vi "MasterAcquisitionFile_IOS.vi"() -> ()   [LabVIEW 2020]
uses:
  <vilib>/vision/driver/IMAQdx.llb/IMAQdx Camera Control Mode.ctl
  <vilib>/vision/driver/IMAQdx.llb/IMAQdx Acquisition Mode.ctl
  <vilib>/userDefined/High Color/IMAQdx.ctl
  <vilib>/vision/driver/IMAQdx.llb/IMAQdx Buffer Number Mode.ctl
  <vilib>/DAQmx/write.llb/DAQmx Write (Digital 1D Wfm NChan NSamp).vi
  <vilib>/DAQmx/read.llb/DAQmx Read (Analog 1D Wfm NChan NSamp).vi
  <vilib>/Waveform/DWDTOps.llb/DWDT Digital to Boolean Array.vi
  <vilib>/DAQmx/create/channels.llb/DAQmx Create Channel (CO-Pulse Generation-Frequency).vi
  <vilib>/DAQmx/configure/timing.llb/DAQmx Timing (Implicit).vi
  <vilib>/DAQmx/create/channels.llb/DAQmx Create Channel (AI-Voltage-Basic).vi
  <vilib>/DAQmx/configure/timing.llb/DAQmx Timing (Sample Clock).vi
  <vilib>/DAQmx/configure/trigger.llb/DAQmx Start Trigger (Digital Edge).vi
  <vilib>/DAQmx/create/channels.llb/DAQmx Create Channel (DO-Digital Output).vi
  <vilib>/Waveform/DWDTOps.llb/DWDT Boolean Array to Digital.vi
  <vilib>/Waveform/DWDTOps.llb/DWDT Uncompress Digital.vi
  <vilib>/DAQmx/miscellaneous.llb/DAQmx Fill In Error Info.vi
  <vilib>/vision/driver/NI_Vision_Acquisition_Software.lvlib
  <resource>/objmgr/imaqdx.rc
  <resource>/objmgr/daqmx.rc
panel:
  out "LED":bool
  out "Auditory":bool
  out "RPad":bool
  out "LPad":bool
  out "Finished":bool
  in  "Generate Stimuli":bool=TRUE
  in  "Sol Stim Parameters":cluster{"Fs":dbl, "Samples":dbl}
  in  "LED Stim Parameters":cluster{"Fs":dbl, "Samples":dbl}
  in  "Sol Duty Cycle (%)":dbl=10.0
  in  "Sol Freq":dbl=1.0
  in  "Sol Dur (s)":dbl=1.0
  in  "LED Duty Cycle (%)":dbl=10.0
  in  "LED Freq":dbl=10.0
  in  "LED Dur (s)":dbl=2.0
  out "Stimulus Order":digitalwaveform[](graph)=[{"t0"=timestamp(0 s since 1904-01-01), "dt"=5e-05, "Y"={"transitions"=[], "data"=array18001000x1[18001000 elements]}}, {"t0"=timestamp(0 s since 1904-01-01), "dt"=5e-05, "Y"={"transitions"=[], "data"=array18001000x1[18001000 elements]}}, {"t0"=timestamp(0 s since 1904-01-01), "dt"=5e-05, "Y"={"transitions"=[], "data"=array18001000x1[18001000 elements]}}, {"t0"=timestamp(0 s since 1904-01-01), "dt"=5e-05, "Y"={"transitions"=[], "data"=array18001000x1[18001000 elements]}}]
  out "Solenoid Stim":digitalwaveform(graph)={"t0"=timestamp(0 s since 1904-01-01), "dt"=5e-05, "Y"={"transitions"=[], "data"=array100000x1[100000 elements]}}
  in  "Trial Offset (s)":dbl=15.0
  in  "Interstim (s)":dbl=30.0
  in  "Right Pad":dbl=1.0
  in  "Left Pad":dbl=1.0
  in  "Auditory":dbl=1.0
  in  "LED":dbl
  out "?":T1(plugin-control)
  out "?":T1(plugin-control)
  out "?":T1(plugin-control)
  out "?":T1(plugin-control)
  in  "stop":bool
  out "CBV Cam":bool=TRUE
  out "Pupil Cam":bool=TRUE
  out "Whisk Cam":bool=TRUE
  out "Web Cam":bool=TRUE
  out "Analog":bool=TRUE
  out "Web Cam Fs":dbl(knob)=29.946097025354362 scale=0.0..200.0
  out "CBV Cam Fs":dbl(knob)=30.0 scale=0.0..200.0
  out "Whisk Cam Fs":dbl(knob)=150.04985044865404 scale=0.0..200.0
  out "Last Whisk\nBuffer 2":u32=16153
  out "Pupil Cam Fs":dbl(knob)=30.00491883915396 scale=0.0..200.0
  out "Dropped 2":u32(slide) caption="Pupil Cam" scale=0.0..99.0
  in  "Exposure Time (microsec)":string="10000"
  out "Dev1 Samples":i32=10769152
  in  "Dev1 Analog Channels":string[](array[string])=["Cortical_LH", "Force_Sensor", "LPadSol", "RPadSol", "AudSol", "Hippocampus", "EMG", "Cortical_RH", "OptoLED"]
  in  "Analog Acquisition":cluster{"Analog Fs":u16}={"Analog Fs"=20000} {"Analog Fs" format="%0.0f"}
  in  "Sampling Rates":T2={"CBV Cam Fs"=30, "Whisk Cam Fs"=150, "Web Cam Fs"=15, "Pupil Cam Fs"=30}
  out "Notes Size":i32=8
  out "Notes Reversed":string[](array[string])=["Experimenter", "Animal ID", "Hemisphere", "Solenoid PSI", "Isoflurane time", "Session ID", "Amplifier Gain", "LED power (mW)"]
  out "Notes Array":string[](array[string])=["LED power (mW)", "Amplifier Gain", "Session ID", "Isoflurane time", "Solenoid PSI", "Hemisphere", "Animal ID", "Experimenter"]
  in  "Notes:":T3={"Experimenter"="Kevin", "Animal ID"="T220", "Hemisphere"="Both", "Solenoid PSI"="10", "Isoflurane time"="1000", "Session ID"="Imaging Session One", "Amplifier Gain"="10000", "LED power (mW)"="10"}
  in  "Target Path":path=path "D:/T220/Imaging Session One - 17 May 2021" caption="Final Save Location"
  out "Dropped":u32(slide) caption="Whisk Cam" scale=0.0..999.0
  out "Filename":string="210517_10_51_27"
  out "CBV Camera":bool
  out "Time Elapsed (Min)":cluster{dbl, dbl}(slide)={15.0, 8.976044850000001} scale=0.0..15.0 scale format="%#_2g"
  in  "Time (min)":dbl(knob)=15.0 min=0.5 max=20.0 step=0.5 scale=0.0..20.0 scale format="%#_2g"
  in  "Temp Path":path=path "D:/LabVIEW Streamed Data" caption="Temporary Path for Streamed Data"
  out "Last CBV\nBuffer":i32=16153
  out "Last Whisk\nBuffer":u32=80766
  # "Dropped Frames"
  # "Stimuli"
  # "LPAD"
  # "RPAD"
  # "AUD"
  # "LED"
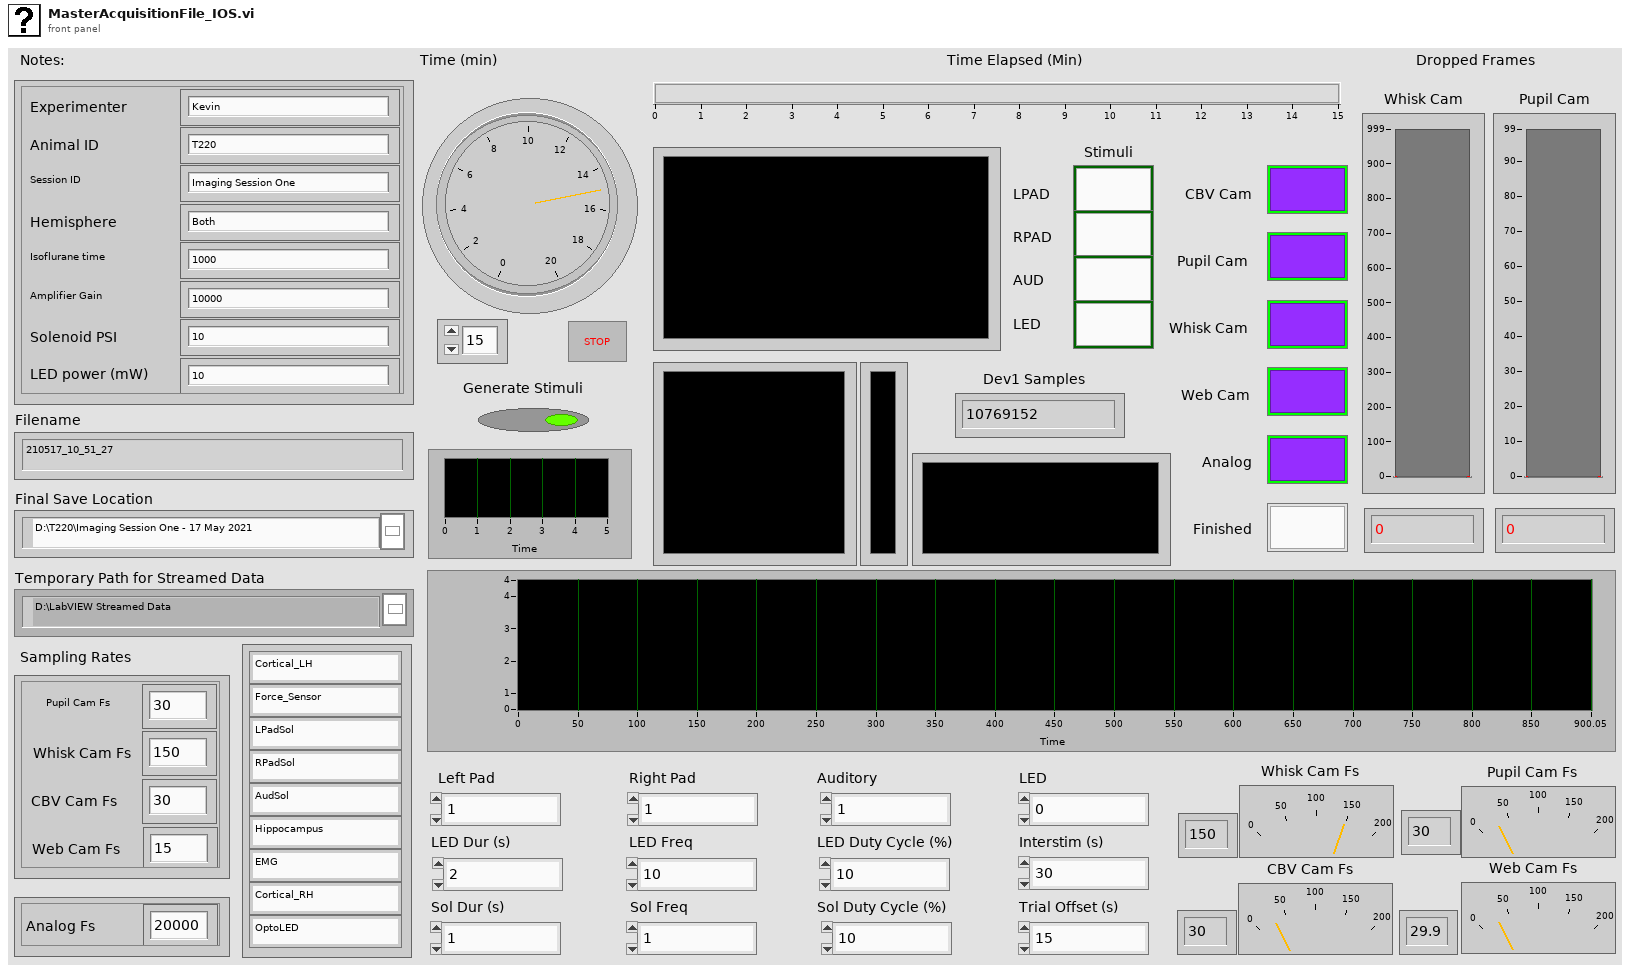
[diagram p1: front panel]
types:
  T1 = typedef "IMAQ Image.ctl" = refnum<image>
  T2 = cluster{"CBV Cam Fs":u16, "Whisk Cam Fs":u16, "Web Cam Fs":u16, "Pupil Cam Fs":u16}
  T3 = cluster{"Experimenter":string, "Animal ID":string, "Hemisphere":string, "Solenoid PSI":string, "Isoflurane time":string, "Session ID":string, "Amplifier Gain":string, "LED power (mW)":string}
  T4 = typedef "IMAQdx.ctl" = refnum<k21>
  T5 = enum16{"open", "replace", "create", "open or create", "replace or create", "replace or create with confirmation"}
  T6 = typedef "Image Type" = u32
  T7 = typedef "NI_Vision_Acquisition_Software.lvlib/IMAQdx Acquisition Mode.ctl" = enum32{"One Shot", "Continuous"}
  T8 = typedef "NI_Vision_Acquisition_Software.lvlib/IMAQdx Camera Control Mode.ctl" = enum32{"Controller", "Listener"}
  T9 = enum16{"open", "open or create", "create or replace", "create", "open (read-only)"}
  T10 = typedef "IMAQ AVI2 Refnum.ctl" = refnum<k20>
  T11 = enum16{"big-endian, network order", "native, host order", "little-endian"}
  T12 = typedef "NI_Vision_Acquisition_Software.lvlib/IMAQdx Buffer Number Mode.ctl" = enum32{"Next", "Last", "Buffer Number", "Every", "Last New"}
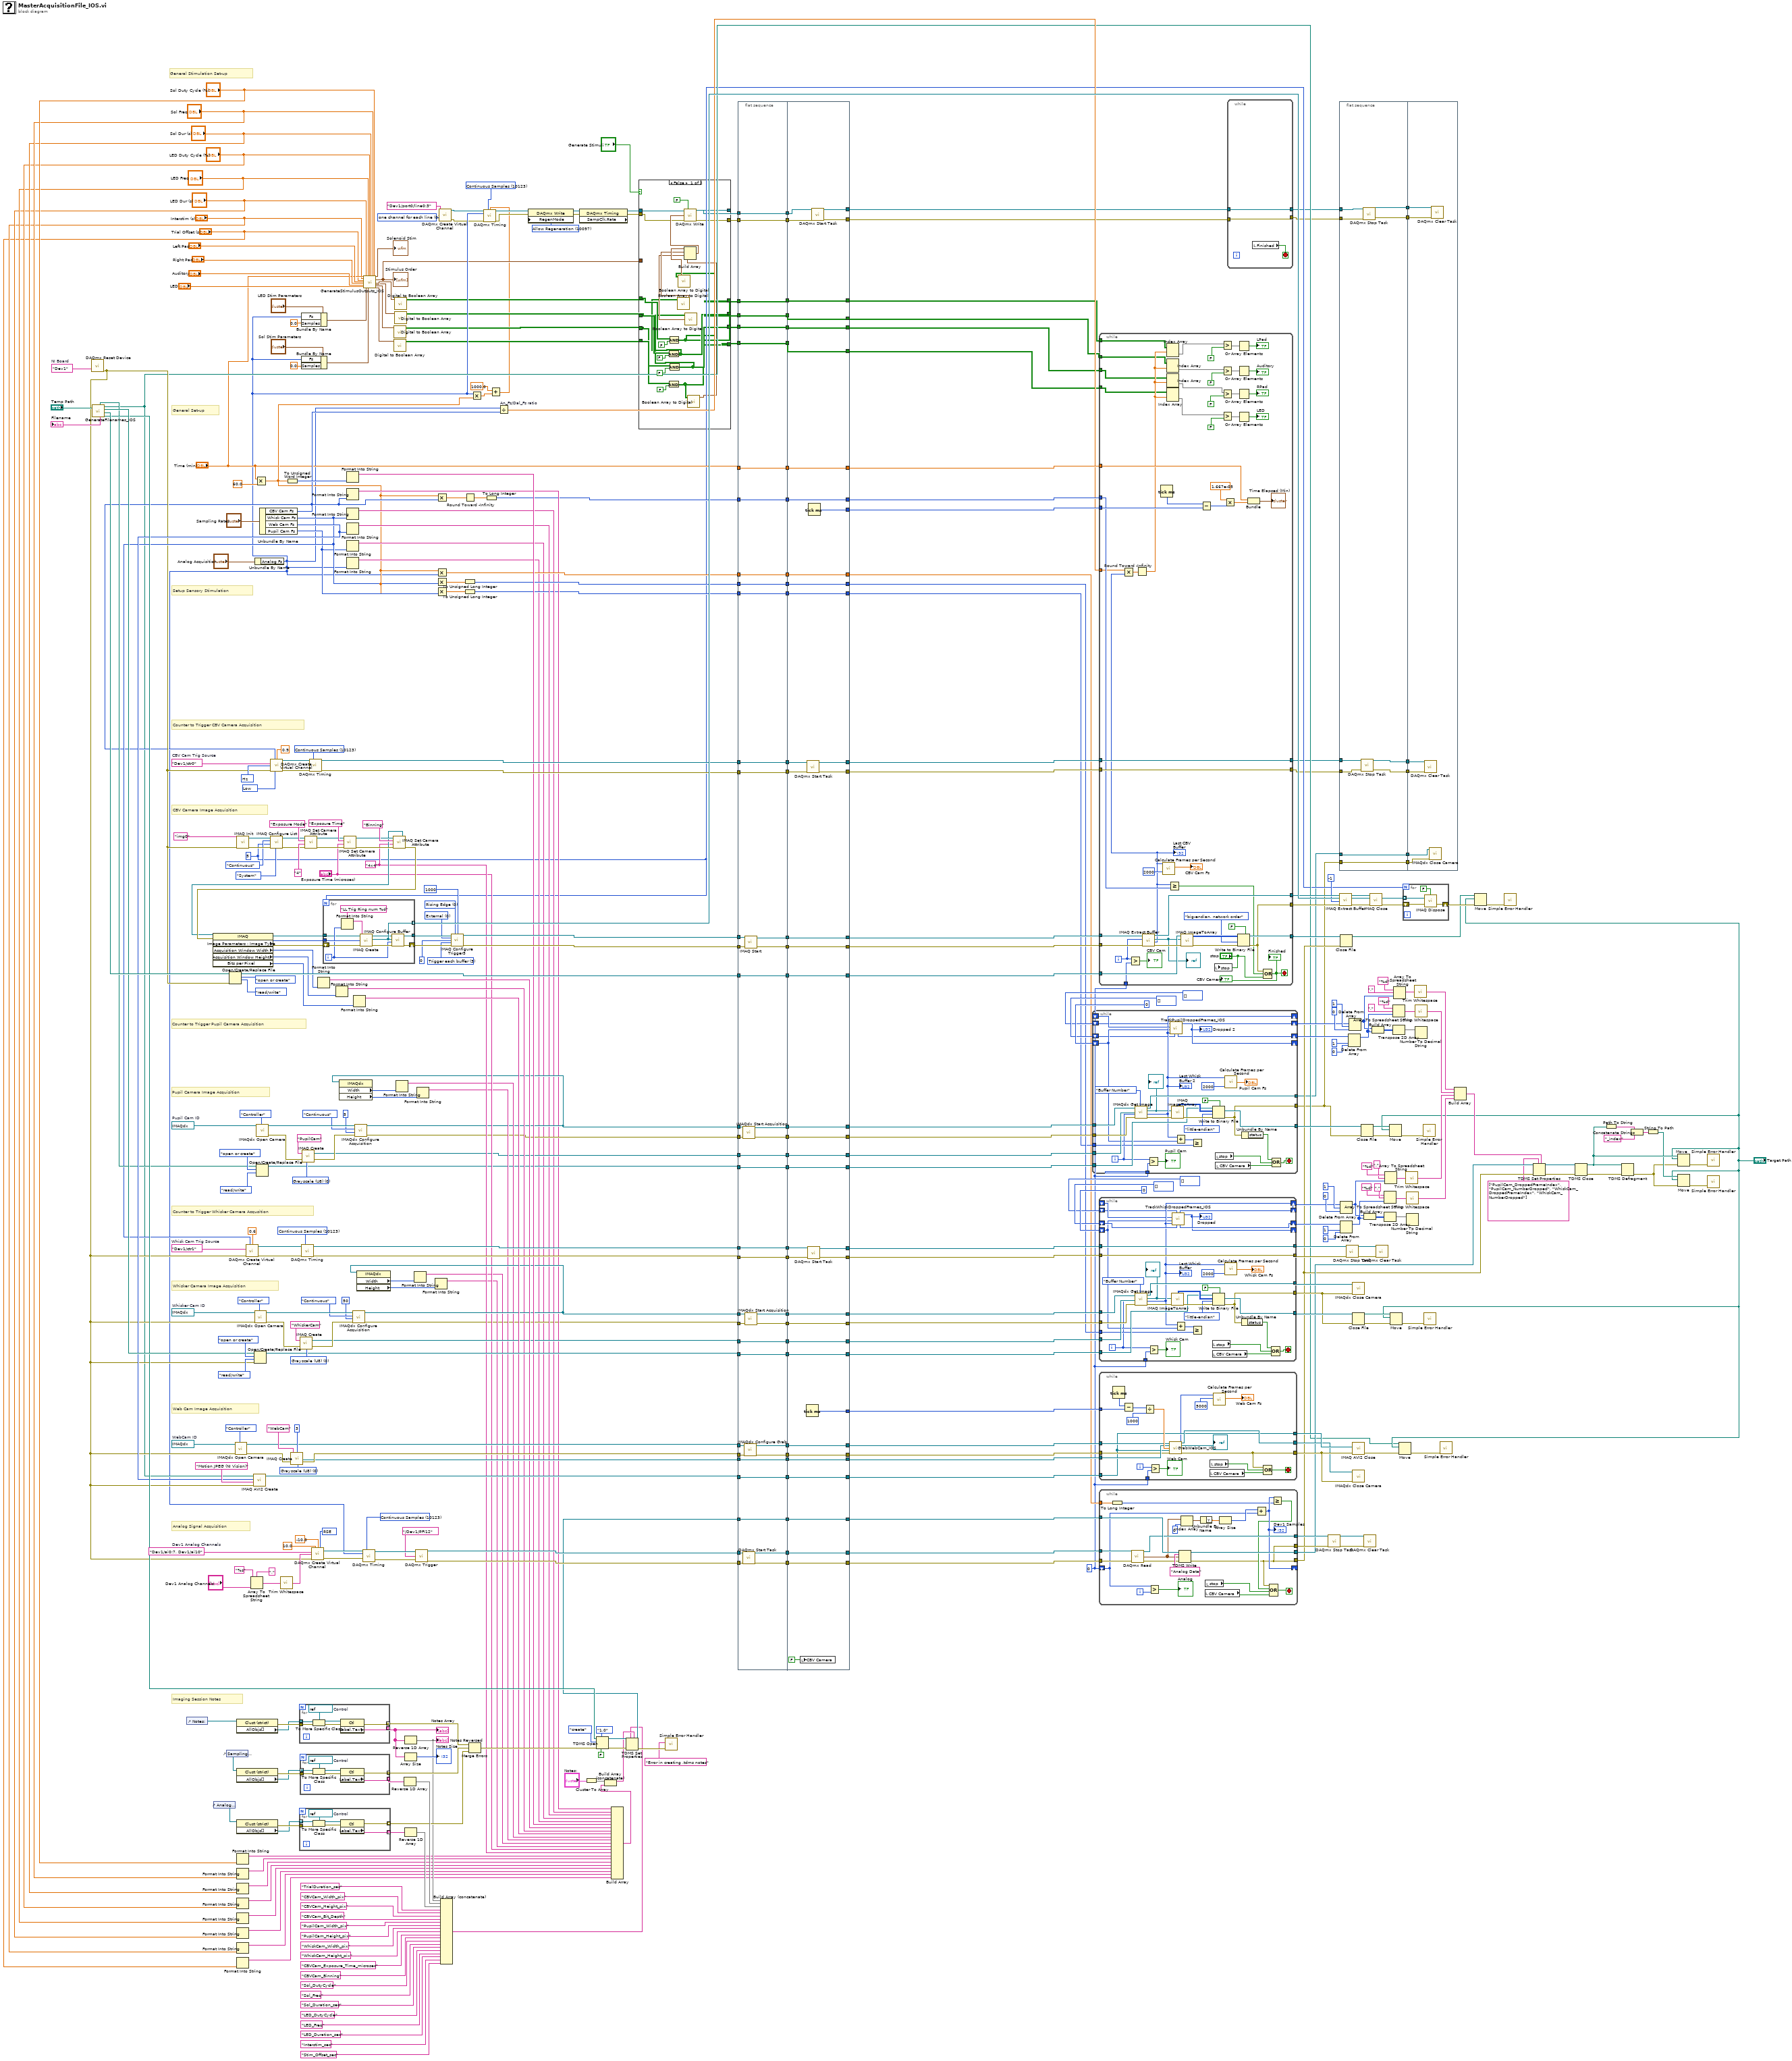
[diagram p0: block diagram]
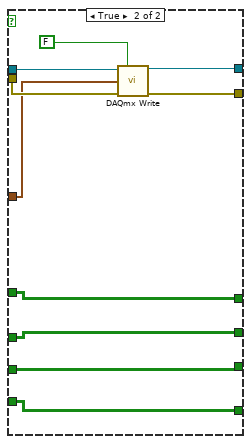
[diagram p2: hidden frame]
diagram:
  w40 = 10097 items=["Allow Regeneration"=10097, "Do Not Allow Regeneration"=10158] ("RegenMode")
  w41 = 10123 items=["Finite Samples"=10178, "Continuous Samples"=10123, "Hardware Timed Single Point"=12522] ("sample mode")
  w44 = 0 items=["one channel for each line", "one channel for all lines"] ("line grouping")
  w258 = tag "Dev1/ai0:7, Dev1/ai10"  # Dev1 Analog Channels
  w261 = T4 "cam0"  # WebCam ID
  w239 = T4 "cam1"  # Whisker Cam ID
  w430 = tag "Dev1/ctr1"  # Whisk Cam Trig Source
  w181 = T4 "cam2"  # Pupil Cam ID
  w5 = tag "Dev1/ctr0"  # CBV Cam Trig Source
  w184 = T6 0 items=["Grayscale (U8)", "Grayscale (I16)", "Grayscale (SGL)", "Complex (CSG)", "RGB (U32)", "HSL (U32)", "RGB (U64)", "Grayscale (U16)"] ("Image Type")
  w171 = "4x4" ("Attribute Value")
  w99 = 0
  w340 = 10123 items=["Finite Samples"=10178, "Continuous Samples"=10123, "Hardware Timed Single Point"=12522] ("sample mode")
  w343 = 10083 items=["default"=-1, "RSE"=10083, "NRSE"=10078, "Differential"=10106, "Pseudodifferential"=12529] ("input terminal configuration")
  w392 = T6 0 items=["Grayscale (U8)", "Grayscale (I16)", "Grayscale (SGL)", "Complex (CSG)", "RGB (U32)", "HSL (U32)", "RGB (U64)", "Grayscale (U16)"] ("Image Type")
  w411 = u32 0 items=["Rising Edge", "Falling Edge"] ("Trigger Polarity")
  w414 = u32 0 items=["External"=0, "RTSI"=1, "ISO In"=2, "Scaled Encoder"=5] ("Trigger Type")
  w405 = tag "Dev1"  # NI Board
  w406 = 10123 items=["Finite Samples"=10178, "Continuous Samples"=10123, "Hardware Timed Single Point"=12522] ("sample mode")
  w409 = 10373 items=["Hz"=10373] ("units")
  w410 = 10214 items=["High"=10192, "Low"=10214] ("idle state")
  w37 = u32 5 ("Number of Buffers")
  w412 = u32 3 items=["Disabled", "Trigger start of acquisition", "Trigger start of each buffer list", "Trigger each buffer", "Trigger each line (linescan)", "Trigger end of acquisition"] ("Action")
  w426 = 10123 items=["Finite Samples"=10178, "Continuous Samples"=10123, "Hardware Timed Single Point"=12522] ("sample mode")
  w433 = T6 0 items=["Grayscale (U8)", "Grayscale (I16)", "Grayscale (SGL)", "Complex (CSG)", "RGB (U32)", "HSL (U32)", "RGB (U64)", "Grayscale (U16)"] ("Image Type")
  # "General Stimulation Set-up"
  # "General Set-up"
  # "Pupil Camera Image Acquisition"
  # "Counter to Trigger Pupil Camera Acquisition"
  # "Whisker Camera Image Acquisition"
  # "Imaging Session Notes"
  # "Setup Sensory Stimulation"
  # "CBV Camera Image Acquisition"
  # "Counter to Trigger CBV Camera Acquisition"
  # "Counter to Trigger Whisker Camera Acqusition"
  # "Web Cam Image Acquisition"
  # "Analog Signal Acquisition"
  n1 = call <vilib>:"DAQmx Reset Device.vi"("device in"=w405) -> ("error out"=w104:errorcluster)  [unwired: 14 in]
  n2 = call "GenerateFilenames_IOS.vi"("path"="Temp Path") -> ("TDMS Path"=w283:path, "Dalsa Path"=w399:path, "Basler Path"=w395:path, "WebCam Path"=w84:path, "Analog file name"=→"Filename":string, "Basler2 Path"=w180:path)  [unwired: 3 in, 2 out]
  n3 = control-ref of="Notes:"() -> (w288:refnum<vi>)
  n4 = control-ref of="Analog Acquisition"() -> (w266:refnum<vi>)
  n5 = control-ref of="Sampling Rates"() -> (w267:refnum<vi>)
  n6 = Open/Create/Replace File(file path (use dialog)=w399, error in=w104, operation (0:open)=T5."open or create", access (0:read/write)=enum16{"read/write", "read-only", "write-only"}."read/write") -> (refnum out=w344:refnum<file>)  [unwired: 2 in, 2 out]
  n7 = call <vilib>:"IMAQdx Open Camera.vi"("Camera Control Mode"=IMAQdx_Camera_Control_Mode."Controller", "error in"=w104, "Session In"=w261) -> ("error out"=w388:errorcluster, "Session Out"=w386:T4)  [unwired: 7 in]
  n8 = property class="Clust (strict)"(reference=w288) -> (error out=w291:errorcluster, "AllObjs[]"=w201:refnum<vi>[])  [unwired: 1 in, 1 out]
  n9 = property class="Clust (strict)"(reference=w267) -> (error out=w286:errorcluster, "AllObjs[]"=w202:refnum<vi>[])  [unwired: 1 in, 1 out]
  n10 = property class="Clust (strict)"(reference=w266) -> (error out=w265:errorcluster, "AllObjs[]"=w200:refnum<vi>[])  [unwired: 1 in, 1 out]
  n11 = call <vilib>:"IMAQ Init.vi"("error in (no error)"=w104, "Interface Name"="img0") -> ("error out"=w424:errorcluster, "IMAQ Session Out"=w425:refnum<k11>)  [unwired: 8 out]
  n12 = Format Into String("Sol Duty Cycle (%)") -> (resulting string=w74:string)  [unwired: 3 in, 1 out]
  n13 = Format Into String("Sol Freq") -> (resulting string=w73:string)  [unwired: 3 in, 1 out]
  n14 = Format Into String("Sol Dur (s)") -> (resulting string=w72:string)  [unwired: 3 in, 1 out]
  n15 = Format Into String("LED Duty Cycle (%)") -> (resulting string=w71:string)  [unwired: 3 in, 1 out]
  n16 = Format Into String("LED Freq") -> (resulting string=w70:string)  [unwired: 3 in, 1 out]
  n17 = Format Into String("LED Dur (s)") -> (resulting string=w69:string)  [unwired: 3 in, 1 out]
  n18 = Format Into String("Interstim (s)") -> (resulting string=w68:string)  [unwired: 3 in, 1 out]
  n19 = Format Into String("Trial Offset (s)") -> (resulting string=w67:string)  [unwired: 3 in, 1 out]
  n20 = Array To Spreadsheet String(delimiter (Tab)=",", array="Dev1 Analog Channels", 3:"%s" ("format string")) -> (spreadsheet string=w255:string)
  n21 = Open/Create/Replace File(file path (use dialog)=w395, error in=w104, operation (0:open)=T5."open or create", access (0:read/write)=enum16{"read/write", "read-only", "write-only"}."read/write") -> (refnum out=w360:refnum<file>)  [unwired: 2 in, 2 out]
  n22 = Unbundle By Name("Analog Acquisition") -> ("Analog Fs"=w57:u16)
  n23 = call <vilib>:"IMAQdx Open Camera.vi"("Camera Control Mode"=IMAQdx_Camera_Control_Mode."Controller", "error in"=w104, "Session In"=w239) -> ("error out"=w436:errorcluster, "Session Out"=w439:T4)  [unwired: 7 in]
  n24 = Multiply(x="Time (min)", y=60.0) -> (x*y=w85:dbl)
  n25 = Open/Create/Replace File(file path (use dialog)=w180, operation (0:open)=T5."open or create", access (0:read/write)=enum16{"read/write", "read-only", "write-only"}."read/write") -> (refnum out=w161:refnum<file>)  [unwired: 3 in, 2 out]
  n26 = call <vilib>:"IMAQdx Open Camera.vi"("Camera Control Mode"=IMAQdx_Camera_Control_Mode."Controller", "Session In"=w181) -> ("error out"=w187:errorcluster, "Session Out"=w190:T4)  [unwired: 8 in]
  n27 = Unbundle By Name("Sampling Rates") -> ("CBV Cam Fs"=w87:u16, "Whisk Cam Fs"=w149:u16, "Web Cam Fs"=w260:u16, "Pupil Cam Fs"=w143:u16)
  n28 = call-poly <vilib>:"DAQmx Create Virtual Channel.vi"("frequency"=w149, "duty cycle"=0.6, "counter"=w430, "error in"=w104) -> ("task out"=w428:refnum<k21>, "error out"=w427:errorcluster)  [unwired: 10 in]
  n29 = call "IMAQ AVI2 Create"("error in (no error)"=w104, "Codec"="Motion JPEG (NI Vision)", "Frames Per Second"=w260, "AVI Path"=w84) -> ("AVI Refnum"=w378:T10)  [unwired: 6 in, 1 out]
  n30 = call-poly <vilib>:"DAQmx Create Virtual Channel.vi"("frequency"=w87, "duty cycle"=0.9, "counter"=w5, "units"=w409, "error in"=w104, "idle state"=w410) -> ("task out"=w408:refnum<k21>, "error out"=w407:errorcluster)  [unwired: 8 in]
  n31 = call <vilib>:"IMAQ Configure List.vi"("Memory Location"=enum16{"System", "Onboard"}."System", "error in (no error)"=w424, "Number of buffers"=w37, "Continuous?"=enum16{"One-Shot", "Continuous"}."Continuous" ("Continuous ?"), "IMAQ Session In"=w425) -> ("error out"=w215:errorcluster, "IMAQ Session Out"=w211:refnum<k11>)  [unwired: 1 in, 4 out]
  n32 = call <vilib>:"Trim Whitespace.vi"("string"=w255) -> ("trimmed string"=w254:string)  [unwired: 1 in]
  n33 = To Unsigned Word Integer(number=w85) -> (unsigned 16bit integer=w250:u16)
  n34 = call "IMAQ Create"("Border Size"=3, "Image Name"="WebCam", "Image Type"=w392, "error in (no error)"=w388) -> ("New Image"=w385:T1, "error out"=w387:errorcluster)  [unwired: 1 in]
  n35 = for {
    tunnel: [w445] -> w290 mode=indexing
    tunnel: w291 -> [w444]
    tunnel: [w442] -> w274 mode=indexing
    tunnel: w201 -> [w441] mode=indexing
    w446 = refnum<vi> refnum  # Control
    n36 = To More Specific Class(target class=w446, reference=w441, error in=w444) -> (specific class reference=w447:refnum<vi>, error out=w443:errorcluster)
    n37 = property class="Ctl"(reference=w447, error in=w443) -> (error out=w442:errorcluster, "Label.Text"=w445:string)  [unwired: 1 out]
  }
  "Notes Array" <- w290
  n38 = for {
    tunnel: [w452] -> w263 mode=indexing
    tunnel: w265 -> [w451]
    tunnel: [w449] -> w264 mode=indexing
    tunnel: w200 -> [w448] mode=indexing
    w453 = refnum<vi> refnum  # Control
    n39 = To More Specific Class(target class=w453, reference=w448, error in=w451) -> (specific class reference=w454:refnum<vi>, error out=w450:errorcluster)
    n40 = property class="Ctl"(reference=w454, error in=w450) -> (error out=w449:errorcluster, "Label.Text"=w452:string)  [unwired: 1 out]
  }
  n41 = call "IMAQ Create"("Image Name"="WhiskerCam", "Image Type"=w433, "error in (no error)"=w436) -> ("New Image"=w237:T1, "error out"=w434:errorcluster)  [unwired: 2 in]
  n42 = for {
    tunnel: [w459] -> w287 mode=indexing
    tunnel: w286 -> [w458]
    tunnel: [w456] -> w273 mode=indexing
    tunnel: w202 -> [w455] mode=indexing
    w460 = refnum<vi> refnum  # Control
    n43 = To More Specific Class(target class=w460, reference=w455, error in=w458) -> (specific class reference=w461:refnum<vi>, error out=w457:errorcluster)
    n44 = property class="Ctl"(reference=w461, error in=w457) -> (error out=w456:errorcluster, "Label.Text"=w459:string)  [unwired: 1 out]
  }
  n45 = Bundle By Name(cluster="LED Stim Parameters", "Fs"=w57, "Samples"=0.0) -> (w92:cluster{"Fs":dbl, "Samples":dbl})
  n46 = Bundle By Name(cluster="Sol Stim Parameters", "Fs"=w57, "Samples"=0.0) -> (w93:cluster{"Fs":dbl, "Samples":dbl})
  n47 = call-poly <vilib>:"DAQmx Timing.vi"("task/channels in"=w428, "sample mode"=w426, "error in"=w427) -> ("task out"=w325:refnum<k21>, "error out"=w323:errorcluster)  [unwired: 11 in]
  n48 = call "IMAQ Create"("Image Name"="PupilCam", "Image Type"=w184, "error in (no error)"=w187) -> ("New Image"=w152:T1, "error out"=w185:errorcluster)  [unwired: 2 in]
  n49 = call <vilib>:"IMAQ Set Camera Attribute.vi"("error in (no error)"=w215, "Attribute Value"="4", "Camera Attribute"="Exposure Mode", "IMAQ Session In"=w211) -> ("error out"=w214:errorcluster, "IMAQ Session Out"=w210:refnum<k11>)  [unwired: 4 in]
  n50 = call-poly <vilib>:"DAQmx Timing.vi"("task/channels in"=w408, "sample mode"=w406, "error in"=w407) -> ("task out"=w329:refnum<k21>, "error out"=w327:errorcluster)  [unwired: 11 in]
  n51 = call-poly <vilib>:"DAQmx Create Virtual Channel.vi"("maximum value"=10.0, "minimum value"=-10.0, "input terminal configuration"=w343, "physical channels"=w258, "name to assign"=w254, "error in"=w104) -> ("task out"=w342:refnum<k21>, "error out"=w341:errorcluster)  [unwired: 8 in]
  n52 = call <vilib>:"IMAQ Set Camera Attribute.vi"("error in (no error)"=w214, "Attribute Value"="Exposure Time (microsec)", "Camera Attribute"="Exposure Time", "IMAQ Session In"=w210) -> ("error out"=w213:errorcluster, "IMAQ Session Out"=w209:refnum<k11>)  [unwired: 4 in]
  n53 = Format Into String(w250) -> (resulting string=w252:string)  [unwired: 3 in, 1 out]
  n54 = Format Into String(w87) -> (resulting string=w147:string)  [unwired: 3 in, 1 out]
  n55 = Format Into String(w149) -> (resulting string=w146:string)  [unwired: 3 in, 1 out]
  n56 = Format Into String(w260) -> (resulting string=w145:string)  [unwired: 3 in, 1 out]
  n57 = Format Into String(w143) -> (resulting string=w106:string)  [unwired: 3 in, 1 out]
  n58 = Format Into String(w57) -> (resulting string=w105:string)  [unwired: 3 in, 1 out]
  n59 = call <vilib>:"IMAQdx Configure Acquisition.vi"("error in"=w434, "Number of Buffers"=u32 50, "Continuous?"=IMAQdx_Acquisition_Mode."Continuous", "Session In"=w439) -> ("error out"=w115:errorcluster, "Session Out"=w238:T4)  [unwired: 6 in]
  n60 = call <vilib>:"IMAQdx Configure Acquisition.vi"("error in"=w185, "Number of Buffers"=u32 5, "Continuous?"=IMAQdx_Acquisition_Mode."Continuous", "Session In"=w190) -> ("error out"=w163:errorcluster, "Session Out"=w153:T4)  [unwired: 6 in]
  n61 = property class="IMAQdx"(reference=w153) -> ("Width"=w179:u32, "Height"=w178:u32)  [unwired: 1 in, 2 out]
  n62 = property class="IMAQdx"(reference=w238) -> ("Width"=w249:u32, "Height"=w248:u32)  [unwired: 1 in, 2 out]
  n63 = call-poly <vilib>:"DAQmx Timing.vi"("task/channels in"=w342, "sample mode"=w340, "rate"=w57, "error in"=w341) -> ("task out"=w198:refnum<k21>, "error out"=w339:errorcluster)  [unwired: 10 in]
  n64 = call "GenerateStimulusOutputs_IOS.vi"("Trial duration (min)"="Time (min)", "Rest duration(s)"="Interstim (s)", "trial offset (s)"="Trial Offset (s)", "Left Pad"="Left Pad", "Right Pad"="Right Pad", "Auditory"="Auditory", "LED"="LED", "LED Stim Duration (s)"="LED Dur (s)", "LED Stim Parameters"=w92, "LED Frequency"="LED Freq", "Sol Stim Parameters"=w93, "LED duty cycle (%)"="LED Duty Cycle (%)", "Sol Stim Duration (s)"="Sol Dur (s)", "Sol Frequency"="Sol Freq", "Sol Duty Cycle (%)"="Sol Duty Cycle (%)") -> ("Solenoid Stim Waveforms"=→"Solenoid Stim":digitalwaveform, "Stimulus Digital Outputs"=w17:digitalwaveform[], "Left Pad Out"=w48:digitalwaveform, "Auditory Out"=w47:digitalwaveform, "Right Pad Out"=w46:digitalwaveform, "LED Out"=w45:digitalwaveform)  [unwired: 7 in]
  "Stimulus Order" <- w17
  n65 = call <vilib>:"IMAQ Set Camera Attribute.vi"("error in (no error)"=w213, "Attribute Value"=w171, "Camera Attribute"="Binning", "IMAQ Session In"=w209) -> ("error out"=w212:errorcluster, "IMAQ Session Out"=w208:refnum<k11>)  [unwired: 4 in]
  n66 = property class="IMAQ"(reference=w208, error in=w212) -> (reference out=w222:refnum<k11>, error out=w221:errorcluster, "Image Parameters : Image Type"=w420:u32, "Acquisition Window Width"=w247:u32, "Acquisition Window Height"=w246:u32, "Bits per Pixel"=w245:u32)
  n67 = Format Into String(w247) -> (resulting string=w244:string)  [unwired: 3 in, 1 out]
  n68 = for {
    N: w37 -> [_]
    tunnel: [w471] -> w416
    tunnel: w420 -> [w469]
    shift-right: [w470] -> w415
    shift-left: w221 -> [w468]
    tunnel: [w463] -> w417 mode=indexing
    tunnel: w222 -> [w462]
    i -> [w464]
    n69 = Format Into String(format string="LL Trig Ring num %d", w464) -> (resulting string=w466:string)  [unwired: 2 in, 1 out]
    n70 = call "IMAQ Create"("Image Name"=w466, "Image Type"=w469, "error in (no error)"=w468) -> ("New Image"=w463:T1, "error out"=w467:errorcluster)  [unwired: 1 in, 1 out]
    n71 = call <vilib>:"IMAQ Configure Buffer.vi"("error in (no error)"=w467, "Buffer Number"=w464, "Image In"=w463, "IMAQ Session In"=w462) -> ("error out"=w470:errorcluster, "IMAQ Session Out"=w471:refnum<k11>)  [unwired: 2 in, 4 out]
  }
  n72 = Format Into String(w246) -> (resulting string=w195:string)  [unwired: 3 in, 1 out]
  n73 = Format Into String(w245) -> (resulting string=w243:string)  [unwired: 3 in, 1 out]
  n74 = call-poly <vilib>:"Digital to Boolean Array.vi"("digital waveform"=w46) -> ("boolean array"=w23:bool[][])  [unwired: 9 in, 1 out]
  n75 = call-poly <vilib>:"Digital to Boolean Array.vi"("digital waveform"=w45) -> ("boolean array"=w22:bool[][])  [unwired: 9 in, 1 out]
  n76 = call-poly <vilib>:"Digital to Boolean Array.vi"("digital waveform"=w48) -> ("boolean array"=w25:bool[][])  [unwired: 9 in, 1 out]
  n77 = call-poly <vilib>:"Digital to Boolean Array.vi"("digital waveform"=w47) -> ("boolean array"=w24:bool[][])  [unwired: 9 in, 1 out]
  n78 = Format Into String(w179) -> (resulting string=w166:string)  [unwired: 3 in, 1 out]
  n79 = Reverse 1D Array(array=w287) -> (reversed array=w277:string[])
  n80 = Reverse 1D Array(array=w290) -> (reversed array=w199:string[])
  "Notes Reversed" <- w199
  n81 = Array Size(array=w290) -> (size(s)=→"Notes Size":i32)
  n82 = Reverse 1D Array(array=w263) -> (reversed array=w262:string[])
  n83 = Format Into String(w249) -> (resulting string=w168:string)  [unwired: 3 in, 1 out]
  n84 = call-poly <vilib>:"DAQmx Trigger.vi"("task/channels in"=w198, "source"=tag "/Dev1/PFI12", "error in"=w339) -> ("task out"=w338:refnum<k21>, "error out"=w337:errorcluster)  [unwired: 11 in]
  n85 = Format Into String(w178) -> (resulting string=w167:string)  [unwired: 3 in, 1 out]
  n86 = Format Into String(w248) -> (resulting string=w169:string)  [unwired: 3 in, 1 out]
  n87 = Multiply(x=w85, y=w87) -> (x*y=w397:dbl)
  n88 = Multiply(x=w85, y=w57) -> (x*y=w226:dbl)
  n89 = Multiply(x=w149, y=w85) -> (x*y=w196:dbl)
  n90 = Multiply(x=w143, y=w85) -> (x*y=w148:dbl)
  n91 = call-poly <vilib>:"DAQmx Create Virtual Channel.vi"("lines"=tag "Dev1/port0/line0:3", "line grouping"=w44) -> ("task out"=w43:refnum<k21>, "error out"=w42:errorcluster)  [unwired: 12 in]
  n92 = Build Array (concatenate)(w199, w277, w262, "TrialDuration_sec", "CBVCam_Width_pix", "CBVCam_Height_pix", "CBVCam_Bit_Depth", "PupilCam_Width_pix", "PupilCam_Height_pix", "WhiskCam_Width_pix", "WhiskCam_Height_pix", "CBVCam_Exposure_Time_microsec" ("element"), "CBVCam_Binning" ("element"), "Sol_DutyCycle", "Sol_Freq", "Sol_Duration_sec", "LED_DutyCycle", "LED_Freq", "LED_Duration_sec", "Interstim_sec", "Stim_Offset_sec") -> (w192:string[])
  n93 = call <vilib>:"IMAQ Configure Trigger3.vi"("IMAQ Session In"=w416, "Polarity"=w411, "Frame timeout (ms)"=u32 1000 ("Frame Timeout (ms)"), "Type"=w414, "Line Number"=u32 0 ("Trigger Line Number"), "Action"=w412, "error in (no error)"=w415) -> ("IMAQ Session Out"=w359:refnum<k11>, "error out"=w358:errorcluster)  [unwired: 2 in, 5 out]
  n94 = To Unsigned Long Integer(number=w196) -> (unsigned 32bit integer=w224:u32)
  n95 = To Unsigned Long Integer(number=w148) -> (unsigned 32bit integer=w144:u32)
  n96 = Round Toward -Infinity(1:w397) -> (0:w396:dbl)
  n97 = Merge Errors(w274, w273, w264) -> (w272:errorcluster)
  n98 = Multiply(x=w57, y=w85) -> (x*y=w16:dbl)
  n99 = To Long Integer(number=w396) -> (32bit integer=w116:i32)
  n100 = Add(x=1000.0, y=w16) -> (x+y=w14:dbl)
  n101 = call-poly <vilib>:"DAQmx Timing.vi"("task/channels in"=w43, "sample mode"=w41, "samples per channel"=w14, "rate"=w57, "error in"=w42) -> ("task out"=w36:refnum<k21>, "error out"=w35:errorcluster)  [unwired: 9 in]
  n102 = Divide "An_Fs/Dal_Fs ratio"(x=w57, y=w87) -> (x/y=w86:dbl)
  n103 = property class="DAQmx Write"(reference=w36, error in=w35, "RegenMode"=w40) -> (reference out=w38:refnum<k21>, error out=w39:errorcluster)
  n104 = property class="DAQmx Timing" props=["SampClk.Rate"](reference=w38, error in=w39) -> (reference out=w33:refnum<k21>, error out=w32:errorcluster)  [unwired: 1 out]
  n105 = Cluster To Array(cluster="Notes:") -> (array=w284:string[])
  n106 = TDMS Open(6:FALSE ("disable buffering? (T)"), 7:enum16{"1.0", "2.0"}."1.0" ("file format version (2.0)"), 8:w272, 10:T9."create" ("operation (0:open)"), 11:w283) -> (0:w278:errorcluster, 3:w279:refnum<k34>)  [unwired: 2 in]
  n107 = Build Array(w147, w146, w145, w106, w105, w252, w244, w195, w243, w166, w167, w168, w169, "Exposure Time (microsec)", w171, w74, w73, w72, w71, w70, w69, w68, w67) -> (w259:string[])
  n108 = Build Array (concatenate)(w284, w259) -> (w276:string[])
  n109 = TDMS Set Properties(5:w276, 7:w192, 8:w278, 11:w279) -> (0:w271:errorcluster, 3:w275:refnum<k34>)  [unwired: 2 in, 2 out]
  n110 = case shown="False" "Generate Stimuli" {
    tunnel: w33 -> [w482 w503]
    tunnel: w32 -> [w481 w502]
    tunnel: [w479 w501] -> w30
    tunnel: [w480 w500] -> w28
    tunnel: w25 -> [w490 w499]
    tunnel: w24 -> [w491 w498]
    tunnel: w23 -> [w492 w497]
    tunnel: w22 -> [w493 w496]
    tunnel: [w474 w499] -> w21
    tunnel: [w475 w498] -> w20
    tunnel: [w476 w497] -> w19
    tunnel: [w472 w496] -> w18
    tunnel: w17 -> [_ w495]
    frame False {
      n111 = Compound Arithmetic op=AND(w491, FALSE) -> (w475:bool[][])
      n112 = Compound Arithmetic op=AND(w493, FALSE) -> (w472:bool[][])
      n113 = Compound Arithmetic op=AND(w490, FALSE) -> (w474:bool[][])
      n114 = Compound Arithmetic op=AND(w492, FALSE) -> (w476:bool[][])
      n115 = call-poly <vilib>:"Boolean Array to Digital.vi"("boolean array"=w475) -> ("digital waveform"=w478:digitalwaveform)  [unwired: 9 in, 1 out]
      n116 = call-poly <vilib>:"Boolean Array to Digital.vi"("boolean array"=w474) -> ("digital waveform"=w484:digitalwaveform)  [unwired: 9 in, 1 out]
      n117 = call-poly <vilib>:"Boolean Array to Digital.vi"("boolean array"=w476) -> ("digital waveform"=w477:digitalwaveform)  [unwired: 9 in, 1 out]
      n118 = call-poly <vilib>:"Boolean Array to Digital.vi"("boolean array"=w472) -> ("digital waveform"=w473:digitalwaveform)  [unwired: 9 in, 1 out]
      n119 = Build Array(w484, w478, w477, w473) -> (w483:digitalwaveform[])
      n120 = call-poly <vilib>:"DAQmx Write.vi"("task/channels in"=w482, "auto start"=FALSE, "data"=w483, "error in"=w481) -> ("task out"=w479:refnum<k21>, "error out"=w480:errorcluster)  [unwired: 9 in, 1 out]
    }
    frame True {
      n121 = call-poly <vilib>:"DAQmx Write.vi"("task/channels in"=w503, "auto start"=FALSE, "data"=w495, "error in"=w502) -> ("task out"=w501:refnum<k21>, "error out"=w500:errorcluster)  [unwired: 9 in, 1 out]
    }
  }
  n122 = call <vilib>:"Simple Error Handler.vi"("error source (\" \")"="Error in creating .tdms notes" ("error source (\" \")"), "error in (no error)"=w271) -> ()  [unwired: 3 in, 5 out]
  n123 = flat-sequence {
    tunnel: w387 -> [w546]
    tunnel: w386 -> [w545]
    tunnel: w385 -> [w544]
    tunnel: [w544] -> w384
    tunnel: [w543] -> w382
    tunnel: [w542] -> w380
    tunnel: w378 -> [w541]
    tunnel: [w541] -> w377
    tunnel: w238 -> [w540]
    tunnel: w115 -> [w539]
    tunnel: [w538] -> w367
    tunnel: [w537] -> w365
    tunnel: [w536] -> w363
    tunnel: w237 -> [w536]
    tunnel: [w535] -> w361
    tunnel: w360 -> [w535]
    tunnel: w359 -> [w534]
    tunnel: w358 -> [w533]
    tunnel: [w532] -> w356
    tunnel: [w531] -> w354
    tunnel: w116 -> [w530]
    tunnel: [w530] -> w350
    tunnel: "Time (min)" -> [w529]
    tunnel: [w529] -> w347
    tunnel: [w528] -> w345
    tunnel: w344 -> [w528]
    tunnel: w338 -> [w527]
    tunnel: w337 -> [w526]
    tunnel: [w525] -> w336
    tunnel: [w524] -> w335
    tunnel: [w523] -> w331
    tunnel: w275 -> [w523]
    tunnel: w329 -> [w522]
    tunnel: [w522] -> w328
    tunnel: w327 -> [w521]
    tunnel: [w521] -> w326
    tunnel: w325 -> [w520]
    tunnel: [w520] -> w324
    tunnel: w323 -> [w519]
    tunnel: [w519] -> w322
    tunnel: w226 -> [w518]
    tunnel: [w518] -> w225
    tunnel: w224 -> [w517]
    tunnel: [w517] -> w223
    tunnel: [w512] -> w165
    tunnel: w153 -> [w513]
    tunnel: [w510] -> w164
    tunnel: w163 -> [w511]
    tunnel: [w516] -> w162
    tunnel: w161 -> [w516]
    tunnel: w152 -> [w515]
    tunnel: [w515] -> w151
    tunnel: w144 -> [w514]
    tunnel: [w514] -> w142
    tunnel: [w509] -> w56
    tunnel: w21 -> [w509]
    tunnel: [w508] -> w55
    tunnel: w20 -> [w508]
    tunnel: [w507] -> w54
    tunnel: w19 -> [w507]
    tunnel: [w506] -> w53
    tunnel: w18 -> [w506]
    tunnel: [w505] -> w31
    tunnel: w30 -> [w505]
    tunnel: [w504] -> w29
    tunnel: w28 -> [w504]
    tunnel: [w588] -> w389
    tunnel: w384 -> [w587]
    tunnel: [w587] -> w383
    tunnel: w382 -> [w586]
    tunnel: [w586] -> w381
    tunnel: w380 -> [w585]
    tunnel: [w585] -> w379
    tunnel: w377 -> [w584]
    tunnel: [w584] -> w376
    tunnel: [w566] -> w373
    tunnel: [w565] -> w371
    tunnel: [w583] -> w368
    tunnel: w367 -> [w583]
    tunnel: [w582] -> w366
    tunnel: w365 -> [w582]
    tunnel: [w581] -> w364
    tunnel: w363 -> [w581]
    tunnel: [w580] -> w362
    tunnel: w361 -> [w580]
    tunnel: [w579] -> w357
    tunnel: w356 -> [w579]
    tunnel: [w578] -> w355
    tunnel: w354 -> [w578]
    tunnel: [w570] -> w353
    tunnel: [w569] -> w352
    tunnel: [w577] -> w351
    tunnel: w350 -> [w576]
    tunnel: [w576] -> w349
    tunnel: [w575] -> w348
    tunnel: w347 -> [w575]
    tunnel: [w574] -> w346
    tunnel: w345 -> [w574]
    tunnel: [w573] -> w333
    tunnel: w336 -> [w573]
    tunnel: [w572] -> w334
    tunnel: w335 -> [w572]
    tunnel: [w571] -> w102
    tunnel: w331 -> [w571]
    tunnel: w328 -> [w568]
    tunnel: w326 -> [w567]
    tunnel: w324 -> [w564]
    tunnel: w322 -> [w563]
    tunnel: w225 -> [w562]
    tunnel: [w562] -> w103
    tunnel: w223 -> [w561]
    tunnel: [w561] -> w141
    tunnel: w165 -> [w559]
    tunnel: w164 -> [w558]
    tunnel: w162 -> [w557]
    tunnel: [w559] -> w157
    tunnel: [w558] -> w156
    tunnel: [w557] -> w155
    tunnel: [w556] -> w150
    tunnel: w151 -> [w556]
    tunnel: [w555] -> w140
    tunnel: w142 -> [w555]
    tunnel: w56 -> [w551]
    tunnel: w55 -> [w554]
    tunnel: w54 -> [w553]
    tunnel: w53 -> [w552]
    tunnel: [w551] -> w52
    tunnel: [w554] -> w51
    tunnel: [w553] -> w50
    tunnel: [w552] -> w49
    tunnel: w31 -> [w550]
    tunnel: w29 -> [w549]
    tunnel: [w548] -> w27
    tunnel: [w547] -> w26
    frame #0 {
      n124 = call <vilib>:"IMAQdx Start Acquisition.vi"("error in"=w511, "Session In"=w513) -> ("error out"=w510:errorcluster, "Session Out"=w512:T4)  [unwired: 8 in]
      n125 = call <vilib>:"DAQmx Start Task.vi"("task/channels in"=w527, "error in"=w526) -> ("task out"=w525:refnum<k21>, "error out"=w524:errorcluster)  [unwired: 12 in]
      n126 = call <vilib>:"IMAQdx Configure Grab.vi"("error in"=w546, "Session In"=w545) -> ("error out"=w542:errorcluster, "Session Out"=w543:T4)  [unwired: 8 in]
      n127 = call <vilib>:"IMAQ Start.vi"("error in (no error)"=w533, "IMAQ Session In"=w534) -> ("error out"=w531:errorcluster, "IMAQ Session Out"=w532:refnum<k11>)  [unwired: 8 out]
      n128 = call <vilib>:"IMAQdx Start Acquisition.vi"("error in"=w539, "Session In"=w540) -> ("error out"=w537:errorcluster, "Session Out"=w538:T4)  [unwired: 8 in]
    }
    frame #1 {
      n129 = local write "CBV Camera"(FALSE ("Finished Acquiring")) -> ()
      n130 = Tick Count (ms)() -> (millisecond timer value=w588:u32)
      n131 = call <vilib>:"DAQmx Start Task.vi"("task/channels in"=w568, "error in"=w567) -> ("task out"=w570:refnum<k21>, "error out"=w569:errorcluster)  [unwired: 12 in]
      n132 = call <vilib>:"DAQmx Start Task.vi"("task/channels in"=w564, "error in"=w563) -> ("task out"=w566:refnum<k21>, "error out"=w565:errorcluster)  [unwired: 12 in]
      n133 = Tick Count (ms)() -> (millisecond timer value=w577:u32)
      n134 = call <vilib>:"DAQmx Start Task.vi"("task/channels in"=w550, "error in"=w549) -> ("task out"=w548:refnum<k21>, "error out"=w547:errorcluster)  [unwired: 12 in]
    }
  }
  n135 = while {
    tunnel: [w603] -> w3
    tunnel: [w604] -> w2
    tunnel: [w613] -> w125
    tunnel: w157 -> [w612]
    tunnel: w156 -> [w611]
    tunnel: w150 -> [w610]
    tunnel: w155 -> [w609]
    shift-right: [w602] -> _
    shift-left: _ -> [w608]
    shift-right: [w607] -> _
    shift-left: u32 0 ("New Lost") -> [w601]
    shift-right: [w606] -> w123
    shift-left: u32[] [] ("NewBuffNum") -> [w597]
    shift-right: [w605] -> w124
    shift-left: u32[] [] ("NewNumLost") -> [w598]
    tunnel: w140 -> [w596]
    tunnel: w99 -> [w594]
    i -> [w589]
    stop <- w599 stop-if-true
    n136 = call <vilib>:"IMAQdx Get Image.vi"("Buffer Number Mode (Next)"=IMAQdx_Buffer_Number_Mode."Buffer Number", "error in"=w611, "Buffer Number In"=w589, "Image In"=w610, "Session In"=w612) -> ("error out"=w620:errorcluster, "Buffer Number Out"=w602:u32, "Image Out"=w591:T1, "Session Out"=w603:T4)  [unwired: 3 in]
    "Last Whisk\nBuffer 2" <- w602
    "?" <- w591
    n137 = Greater?(x=w589, y=w594) -> (0:→"Pupil Cam":bool)
    n138 = call "TrackPupilDroppedFrames_IOS.vi"("NumLost"=w598, "BuffNum"=w597, "Curr Buffer"=w602, "Prev Lost"=w601, "Prev Buffer"=w608) -> ("New Lost"=w607:u32, "NewNumLost"=w605:u32[], "NewBuffNum"=w606:u32[])  [unwired: 4 in]
    "Dropped 2" <- w607
    n139 = call "IMAQ ImageToArray"("error in (no error)"=w620, "Image"=w591) -> ("error out"=w619:errorcluster, "Image Pixels (U8)"=w618:u8[][])  [unwired: 2 in, 3 out]
    n140 = Add(x=w602, y=w601) -> (x+y=w600:u32)
    n141 = Greater Or Equal?(x=w600, y=w596) -> ()  [unwired: 1 out]
    n142 = Write to Binary File(file (use dialog)=w609, data=w618, error in=w619, 5:FALSE ("prepend array or string size? (T)"), 9:T11."little-endian" ("byte order (0:big-endian, network order)")) -> (refnum out=w613:refnum<file>, error out=w604:errorcluster)  [unwired: 1 in, 1 out]
    n143 = local read "stop"() -> (w593:bool)
    n144 = local read "CBV Camera"() -> (w592:bool)
    n145 = call <vilib>:"Calculate Frames per Second.vi"("Update Interval (ms)"=u32 2000, "Buffer Number"=w602) -> ("Processed Frames/s"=→"Pupil Cam Fs":dbl)  [unwired: 7 in, 2 out]
    n146 = Unbundle By Name(w604) -> ("status"=w590:bool)
    n147 = Compound Arithmetic op=OR(w590, w593, w592) -> (w599:bool)
  }
  n148 = while {
    tunnel: w357 -> [w674]
    tunnel: w355 -> [w675]
    tunnel: [w657] -> w401
    tunnel: [w655] -> w402
    tunnel: [w669] -> w400
    tunnel: [w664] -> w9
    tunnel: w353 -> [w664]
    tunnel: [w663] -> w8
    tunnel: w352 -> [w663]
    tunnel: w351 -> [w662]
    tunnel: w349 -> [w661]
    tunnel: w348 -> [w660]
    tunnel: w346 -> [w654]
    tunnel: w99 -> [w649]
    tunnel: w86 -> [w644]
    tunnel: w52 -> [w632]
    tunnel: w51 -> [w633]
    tunnel: w50 -> [w627]
    tunnel: w49 -> [w624]
    i -> [w650]
    stop <- w643 stop-if-true
    n149 = Greater?(x=w650, y=w649) -> (0:→"CBV Cam":bool)
    n150 = call <vilib>:"IMAQ Extract Buffer.vi"("error in (no error)"=w675, "Buffer to extract"=w650, "IMAQ Session In"=w674) -> ("error out"=w668:errorcluster, "Buffer Number"=w645:i32, "Image Out"=w647:T1, "IMAQ Session Out"=w655:refnum<k11>)  [unwired: 5 out]
    "Last CBV\nBuffer" <- w645
    "?" <- w647
    n151 = Multiply(x=w644, y=w645) -> (x*y=w646:dbl)
    n152 = Round Toward -Infinity(1:w646) -> (0:w638:dbl)
    n153 = Tick Count (ms)() -> (millisecond timer value=w667:u32)
    n154 = call <vilib>:"Calculate Frames per Second.vi"("Update Interval (ms)"=u32 2000, "Buffer Number"=w645) -> ("Processed Frames/s"=→"CBV Cam Fs":dbl)  [unwired: 7 in, 2 out]
    n155 = Index Array(array=w632, index (row)=w638) -> (element=w631:bool[])  [unwired: 1 in]
    n156 = Index Array(array=w633, index (row)=w638) -> (element=w629:bool[])  [unwired: 1 in]
    n157 = Index Array(array=w627, index (row)=w638) -> (element=w626:bool[])  [unwired: 1 in]
    n158 = Index Array(array=w624, index (row)=w638) -> (element=w623:bool[])  [unwired: 1 in]
    n159 = Greater Or Equal?(x=w645, y=w661) -> (x >= y?=w653:bool)
    n160 = call "IMAQ ImageToArray"("error in (no error)"=w668, "Image"=w647) -> ("error out"=w673:errorcluster, "Image Pixels (I16)"=w672:i16[][])  [unwired: 2 in, 3 out]
    n161 = Subtract(x=w667, y=w662) -> (x-y=w666:u32)
    n162 = local write "stop"("stop") -> ()
    n163 = Greater?(x=w631, y=FALSE ("Boolean")) -> (0:w630:bool[])
    n164 = Greater?(x=w629, y=FALSE ("Boolean")) -> (0:w628:bool[])
    n165 = Greater?(x=w626, y=FALSE ("Boolean")) -> (0:w625:bool[])
    n166 = Greater?(x=w623, y=FALSE ("Boolean")) -> (0:w622:bool[])
    n167 = Multiply(x=w666, y=1.667e-05) -> (x*y=w665:dbl)
    n168 = Or Array Elements(Boolean array=w630) -> (logical OR=→"LPad":bool)
    n169 = Or Array Elements(Boolean array=w628) -> (logical OR=→"Auditory":bool)
    n170 = Or Array Elements(Boolean array=w625) -> (logical OR=→"RPad":bool)
    n171 = Or Array Elements(Boolean array=w622) -> (logical OR=→"LED":bool)
    n172 = Write to Binary File(file (use dialog)=w654, data=w672, error in=w673, 5:FALSE ("prepend array or string size? (T)"), 9:T11."big-endian, network order" ("byte order (0:big-endian, network order)")) -> (refnum out=w669:refnum<file>, error out=w657:errorcluster)  [unwired: 1 in, 1 out]
    n173 = Bundle("Time (min)"=w660, w665) -> (→"Time Elapsed (Min)":cluster{"Time (min)":dbl, dbl})  [unwired: 1 in]
    n174 = Compound Arithmetic op=OR(w657, w653, "stop") -> (w643:bool)
    "CBV Camera" <- w643
    "Finished" <- w643
  }
  n175 = while {
    tunnel: w373 -> [w702]
    tunnel: [w703] -> w372
    tunnel: w371 -> [w703]
    tunnel: [w702] -> w370
    tunnel: [w695] -> w235
    tunnel: [w696] -> w292
    tunnel: [w701] -> w369
    tunnel: w368 -> [w700]
    tunnel: w366 -> [w699]
    tunnel: w364 -> [w698]
    tunnel: w362 -> [w697]
    shift-right: [w686] -> _
    shift-left: _ -> [w684]
    shift-right: [w681] -> _
    shift-left: u32 0 ("New Lost") -> [w685]
    shift-right: [w682] -> w227
    shift-left: u32[] [] ("NewBuffNum") -> [w683]
    shift-right: [w688] -> w316
    shift-left: u32[] [] ("NewNumLost") -> [w687]
    tunnel: w141 -> [w693]
    tunnel: w99 -> [w689]
    i -> [w676]
    stop <- w692 stop-if-true
    n176 = call <vilib>:"IMAQdx Get Image.vi"("Buffer Number Mode (Next)"=IMAQdx_Buffer_Number_Mode."Buffer Number", "error in"=w699, "Buffer Number In"=w676, "Image In"=w698, "Session In"=w700) -> ("error out"=w709:errorcluster, "Buffer Number Out"=w686:u32, "Image Out"=w678:T1, "Session Out"=w695:T4)  [unwired: 3 in]
    "Last Whisk\nBuffer" <- w686
    "?" <- w678
    n177 = Greater?(x=w676, y=w689) -> (0:→"Whisk Cam":bool)
    n178 = call "IMAQ ImageToArray"("error in (no error)"=w709, "Image"=w678) -> ("error out"=w708:errorcluster, "Image Pixels (U8)"=w707:u8[][])  [unwired: 2 in, 3 out]
    n179 = call "TrackWhiskDroppedFrames_IOS.vi"("NumLost"=w687, "BuffNum"=w683, "Curr Buffer"=w686, "Prev Lost"=w685, "Prev Buffer"=w684) -> ("New Lost"=w681:u32, "NewNumLost"=w688:u32[], "NewBuffNum"=w682:u32[])  [unwired: 4 in]
    "Dropped" <- w681
    n180 = Add(x=w686, y=w685) -> (x+y=w694:u32)
    n181 = Greater Or Equal?(x=w694, y=w693) -> ()  [unwired: 1 out]
    n182 = Write to Binary File(file (use dialog)=w697, data=w707, error in=w708, 5:FALSE ("prepend array or string size? (T)"), 9:T11."little-endian" ("byte order (0:big-endian, network order)")) -> (refnum out=w701:refnum<file>, error out=w696:errorcluster)  [unwired: 1 in, 1 out]
    n183 = local read "stop"() -> (w680:bool)
    n184 = local read "CBV Camera"() -> (w679:bool)
    n185 = call <vilib>:"Calculate Frames per Second.vi"("Update Interval (ms)"=u32 2000, "Buffer Number"=w686) -> ("Processed Frames/s"=→"Whisk Cam Fs":dbl)  [unwired: 7 in, 2 out]
    n186 = Unbundle By Name(w696) -> ("status"=w677:bool)
    n187 = Compound Arithmetic op=OR(w677, w680, w679) -> (w692:bool)
  }
  n188 = while {
    tunnel: w389 -> [w727]
    tunnel: w383 -> [w725]
    tunnel: w381 -> [w724]
    tunnel: w379 -> [w723]
    tunnel: w376 -> [w721]
    tunnel: [w722] -> w154
    tunnel: [w713] -> w374
    tunnel: [w721] -> w375
    tunnel: w99 -> [w716]
    i -> [w717]
    stop <- w714 stop-if-true
    n189 = Tick Count (ms)() -> (millisecond timer value=w729:u32)
    n190 = Subtract(x=w729, y=w727) -> (x-y=w730:u32)
    n191 = Divide(x=w730, y=u32 1000) -> (x/y=w726:dbl)
    n192 = Greater?(x=w717, y=w716) -> (0:→"Web Cam":bool)
    n193 = call "GrabWebCam_IOS.vi"("Session In"=w724, "Image In"=w725, "Trial Time"=w726, "AVI Refnum"=w721, "error in"=w723) -> ("Session Out"=w722:T4, "WebCam Img Out"=→"?":T1, "Buffer Number Out"=w720:u32, "error out"=w713:errorcluster)  [unwired: 7 in]
    n194 = local read "CBV Camera"() -> (w715:bool)
    n195 = local read "stop"() -> (w712:bool)
    n196 = call <vilib>:"Calculate Frames per Second.vi"("Update Interval (ms)"=u32 5000, "Buffer Number"=w720) -> ("Processed Frames/s"=→"Web Cam Fs":dbl)  [unwired: 7 in, 2 out]
    n197 = Compound Arithmetic op=OR(w713, w712, w715) -> (w714:bool)
  }
  n198 = while {
    tunnel: w334 -> [w754]
    tunnel: w333 -> [w753]
    tunnel: w102 -> [w752]
    tunnel: [w751] -> w118
    tunnel: [w740] -> w117
    tunnel: [w750] -> w330
    shift-right: [w744] -> _
    shift-left: w99 -> [w735]
    tunnel: [w740] -> w193
    tunnel: w103 -> [w738]
    i -> [w736]
    stop <- w741 stop-if-true
    n199 = To Long Integer(number=w738) -> (32bit integer=w739:i32)
    n200 = call-poly <vilib>:"DAQmx Read.vi"("task/channels in"=w753, "error in"=w754) -> ("task out"=w750:refnum<k21>, "data"=w732:waveform(dbl)[], "error out"=w743:errorcluster)  [unwired: 11 in]
    n201 = Greater?(x=w735, y=w736) -> (0:→"Analog":bool)
    n202 = TDMS Write(0:w752, 5:"Analog Data" ("group name in (Untitled)"), 9:w732, 11:w743) -> (4:w751:refnum<k34>, 15:w740:errorcluster)  [unwired: 2 in, 2 out]
    n203 = Index Array(array=w732, index=0) -> (element=w747:waveform(dbl))
    n204 = Unbundle By Name(w747) -> ("Y"=w746:dbl[])
    n205 = local read "CBV Camera"() -> (w734:bool)
    n206 = local read "stop"() -> (w733:bool)
    n207 = Array Size(array=w746) -> (size(s)=w745:i32)
    n208 = Add(x=w745, y=w735) -> (x+y=w744:i32)
    "Dev1 Samples" <- w744
    n209 = Greater Or Equal?(x=w744, y=w739) -> (x >= y?=w742:bool)
    n210 = Compound Arithmetic op=OR(w740, w742, w733, w734) -> (w741:bool)
  }
  n211 = while {
    tunnel: w27 -> [w755]
    tunnel: [w756] -> w12
    tunnel: w26 -> [w756]
    tunnel: [w755] -> w13
    stop <- w757 stop-if-true
    n212 = local read "Finished"() -> (w757:bool)
  }
  n213 = call <vilib>:"DAQmx Stop Task.vi"("task/channels in"=w330, "error in"=w193) -> ("task out"=w294:refnum<k21>, "error out"=w293:errorcluster)  [unwired: 12 in]
  n214 = flat-sequence {
    tunnel: w13 -> [w767]
    tunnel: w12 -> [w766]
    tunnel: [w765] -> w11
    tunnel: [w764] -> w10
    tunnel: w9 -> [w763]
    tunnel: w8 -> [w762]
    tunnel: [w761] -> w7
    tunnel: [w760] -> w6
    tunnel: [w759] -> w4
    tunnel: w3 -> [w759]
    tunnel: w2 -> [w758]
    tunnel: [w758] -> w1
    tunnel: w11 -> [w773]
    tunnel: w10 -> [w772]
    tunnel: w7 -> [w771]
    tunnel: w6 -> [w770]
    tunnel: w4 -> [w769]
    tunnel: w1 -> [w768]
    frame #0 {
      n215 = call <vilib>:"DAQmx Stop Task.vi"("task/channels in"=w763, "error in"=w762) -> ("task out"=w761:refnum<k21>, "error out"=w760:errorcluster)  [unwired: 12 in]
      n216 = call <vilib>:"DAQmx Stop Task.vi"("task/channels in"=w767, "error in"=w766) -> ("task out"=w765:refnum<k21>, "error out"=w764:errorcluster)  [unwired: 12 in]
    }
    frame #1 {
      n217 = call <vilib>:"DAQmx Clear Task.vi"("task in"=w771, "error in"=w770) -> ()  [unwired: 13 in, 1 out]
      n218 = call <vilib>:"IMAQdx Close Camera.vi"("error in"=w768, "Session In"=w769) -> ()  [unwired: 9 in, 1 out]
      n219 = call <vilib>:"DAQmx Clear Task.vi"("task in"=w773, "error in"=w772) -> ()  [unwired: 13 in, 1 out]
    }
  }
  n220 = call <vilib>:"IMAQ Extract Buffer.vi"("error in (no error)"=w401, "Buffer to extract"=-1, "IMAQ Session In"=w402) -> ("error out"=w422:errorcluster, "IMAQ Session Out"=w421:refnum<k11>)  [unwired: 7 out]
  n221 = Close File(refnum=w400, error in=w117) -> (path=w310:path)  [unwired: 1 out]
  n222 = Delete From Array(array=w227, length=1, index=0) -> (array with subset deleted=w204:u32[])  [unwired: 1 out]
  n223 = Delete From Array(array=w316, length=1, index=0) -> (array with subset deleted=w205:u32[])  [unwired: 1 out]
  n224 = call <vilib>:"DAQmx Stop Task.vi"("task/channels in"=w370, "error in"=w372) -> ("task out"=w113:refnum<k21>, "error out"=w114:errorcluster)  [unwired: 12 in]
  n225 = Delete From Array(array=w124, length=1, index=0) -> (array with subset deleted=w127:u32[])  [unwired: 1 out]
  n226 = Delete From Array(array=w123, length=1, index=0) -> (array with subset deleted=w126:u32[])  [unwired: 1 out]
  n227 = call <vilib>:"IMAQdx Close Camera.vi"("error in"=w292, "Session In"=w235) -> ()  [unwired: 9 in, 1 out]
  n228 = Close File(refnum=w369, error in=w292) -> (path=w308:path, error out=w307:errorcluster)
  n229 = call "IMAQ AVI2 Close"("error in (no error)"=w374, "AVI Refnum"=w375) -> ("error out"=w309:errorcluster)  [unwired: 9 in]
  n230 = call <vilib>:"IMAQdx Close Camera.vi"("error in"=w374, "Session In"=w154) -> ()  [unwired: 9 in, 1 out]
  n231 = Close File(refnum=w125, error in=w2) -> (path=w120:path, error out=w119:errorcluster)
  n232 = Build Array(w204, w205) -> (w207:u32[][])
  n233 = call <vilib>:"DAQmx Clear Task.vi"("task in"=w294, "error in"=w293) -> ()  [unwired: 13 in, 1 out]
  n234 = call <vilib>:"IMAQ Close.vi"("error in (no error)"=w422, "IMAQ Session In"=w421) -> ("error out"=w423:errorcluster)  [unwired: 9 out]
  n235 = Build Array(w126, w127) -> (w129:u32[][])
  n236 = call <vilib>:"DAQmx Clear Task.vi"("task in"=w113, "error in"=w114) -> ()  [unwired: 13 in, 1 out]
  n237 = Array To Spreadsheet String(delimiter (Tab)=",", array=w205, 3:"%d" ("format string")) -> (spreadsheet string=w228:string)
  n238 = Transpose 2D Array(2D array=w207) -> (transposed array=w206:u32[][])
  n239 = Array To Spreadsheet String(delimiter (Tab)=",", array=w204, 3:"%d" ("format string")) -> (spreadsheet string=w229:string)
  n240 = Move(source path=w120, error in=w119, 10:"Target Path") -> (error out=w121:errorcluster)  [unwired: 2 in, 2 out]
  n241 = Move(source path=w308, error in=w307, 10:"Target Path") -> (error out=w305:errorcluster)  [unwired: 2 in, 2 out]
  n242 = Array To Spreadsheet String(delimiter (Tab)=",", array=w127, 3:"%d" ("format string")) -> (spreadsheet string=w130:string)
  n243 = Transpose 2D Array(2D array=w129) -> (transposed array=w128:u32[][])
  n244 = Array To Spreadsheet String(delimiter (Tab)=",", array=w126, 3:"%d" ("format string")) -> (spreadsheet string=w131:string)
  n245 = Move(source path=w84, error in=w309, 10:"Target Path") -> (error out=w304:errorcluster)  [unwired: 2 in, 2 out]
  n246 = for {
    N: w37 -> [_]
    tunnel: w417 -> [w777] mode=indexing
    shift-right: [w775] -> w312
    shift-left: w423 -> [w776]
    n247 = call "IMAQ Dispose"("All Images? (No)"=FALSE, "Image"=w777, "error in (no error)"=w776) -> ("error out"=w775:errorcluster)  [unwired: 3 out]
  }
  n248 = call <vilib>:"Trim Whitespace.vi"("string"=w229) -> ("trimmed string"=w109:string)  [unwired: 1 in]
  n249 = call <vilib>:"Trim Whitespace.vi"("string"=w228) -> ("trimmed string"=w108:string)  [unwired: 1 in]
  n250 = Number To Decimal String(number=w206) -> ()  [unwired: 1 in, 1 out]
  n251 = call <vilib>:"Trim Whitespace.vi"("string"=w131) -> ("trimmed string"=w110:string)  [unwired: 1 in]
  n252 = call <vilib>:"Trim Whitespace.vi"("string"=w130) -> ("trimmed string"=w111:string)  [unwired: 1 in]
  n253 = Number To Decimal String(number=w128) -> ()  [unwired: 1 in, 1 out]
  n254 = call <vilib>:"Simple Error Handler.vi"("error in (no error)"=w121) -> ()  [unwired: 1 in, 8 out]
  n255 = call <vilib>:"Simple Error Handler.vi"("error in (no error)"=w305) -> ()  [unwired: 1 in, 8 out]
  n256 = call <vilib>:"Simple Error Handler.vi"("error in (no error)"=w304) -> ()  [unwired: 1 in, 8 out]
  n257 = Build Array(w110, w111, w109, w108) -> (w107:string[])
  n258 = Move(source path=w310, error in=w312, 10:"Target Path") -> (error out=w311:errorcluster)  [unwired: 2 in, 2 out]
  n259 = call <vilib>:"Simple Error Handler.vi"("error in (no error)"=w311) -> ()  [unwired: 1 in, 8 out]
  n260 = TDMS Set Properties(5:w107, 7:string[] ["PupilCam_DroppedFrameIndex", "PupilCam_NumberDropped", "WhiskCam_DroppedFrameIndex", "WhiskCam_NumberDropped"] ("channel name(s) in (Untitled)"), 8:w117, 11:w118) -> (0:w236:errorcluster, 3:w234:refnum<k34>)  [unwired: 2 in, 2 out]
  n261 = TDMS Close(8:w236, 11:w234) -> (0:w313:errorcluster, 3:w301:path)
  n262 = Path To String(path=w301) -> (string=w303:string)
  n263 = TDMS Defragment(4:w313, 7:w301) -> (0:w298:errorcluster)
  n264 = Concatenate Strings(w303, "_index" ("string")) -> (w300:string)
  n265 = String To Path(string=w300) -> (path=w299:path)
  n266 = Move(source path=w301, error in=w298, 10:"Target Path") -> (error out=w306:errorcluster)  [unwired: 2 in, 2 out]
  n267 = Move(source path=w299, error in=w298, 10:"Target Path") -> (error out=w122:errorcluster)  [unwired: 2 in, 2 out]
  n268 = call <vilib>:"Simple Error Handler.vi"("error in (no error)"=w306) -> ()  [unwired: 1 in, 8 out]
  n269 = call <vilib>:"Simple Error Handler.vi"("error in (no error)"=w122) -> ()  [unwired: 1 in, 8 out]
